vi "Waveform Shift 2 channels.vi"(8 "Trigger Info":cluster{"Trigger":bool, "Trig Offset":u8}, 9 "Input Valid":bool, 11 "Input Data":i16[](array[numeric])=[0, 0, 0, 0, 0, 0, 0, 0]) -> (0 "Trig Info":cluster{"Trigger":bool, "Trig Offset":u8}, 1 "Output Valid":bool, 3 "Shifted Output Data":i16[](array[numeric]), 4 "Trig Num":u8)   [LabVIEW 2012]
uses:
  <vilib>/rvi/FXPMathLib/basic elements/FxpDiscreteDelay/XNode/nifxpmath_DiscreteDelay.xnode
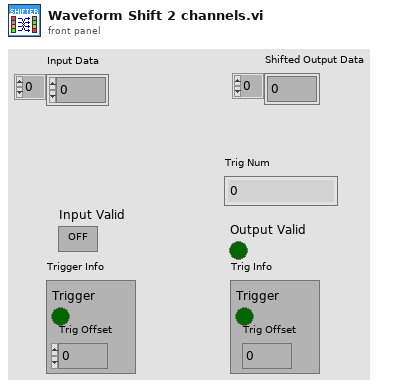
[diagram p1: front panel]
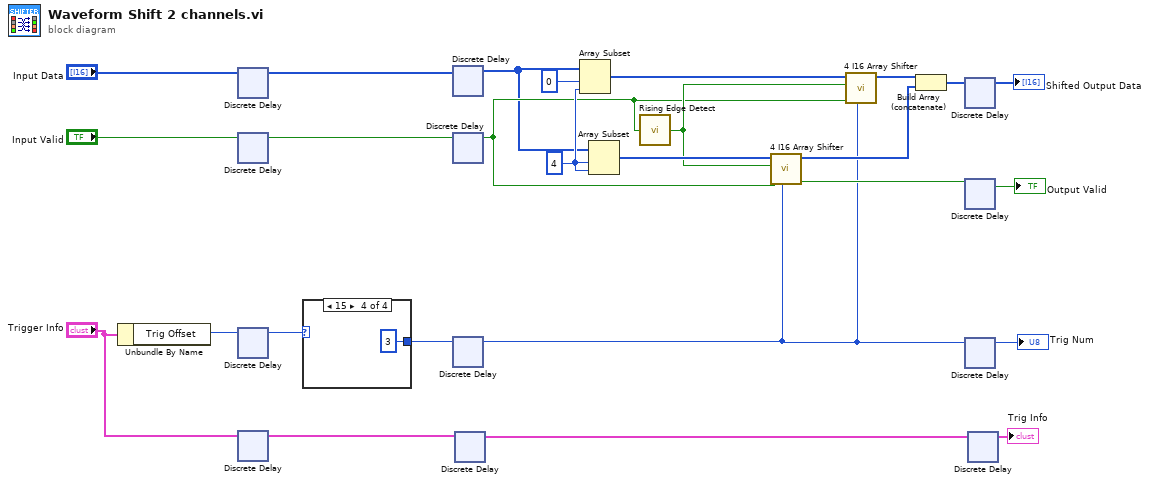
[diagram p0: block diagram]
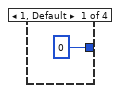
[diagram p2: hidden frame]
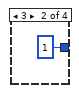
[diagram p3: hidden frame]
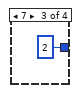
[diagram p4: hidden frame]
diagram:
  w26 = 4 ("index")
  n1 = Unbundle By Name("Trigger Info") -> ("Trig Offset"=w10:u8)
  n2 = xnode "Discrete Delay"("D"="Input Data") -> ("Q"=w6:i16[])
  n3 = xnode "Discrete Delay"("D"="Input Valid") -> ("Q"=w7:bool)
  n4 = xnode "Discrete Delay"("D"=w10) -> ("Q"=w3:u8)
  n5 = xnode "Discrete Delay"("D"="Trigger Info") -> ("Q"=w5:cluster{"Trigger":bool, "Trig Offset":u8})
  n6 = case shown="15" w3 {
    tunnel: [u8 0 u8 1 u8 2 u8 3] -> w2
    frame 1, Default {
    }
    frame 3 {
    }
    frame 7 {
    }
    frame 15 {
    }
  }
  n7 = xnode "Discrete Delay"("D"=w6) -> ("Q"=w17:i16[])
  n8 = xnode "Discrete Delay"("D"=w7) -> ("Q"=w18:bool)
  n9 = xnode "Discrete Delay"("D"=w2) -> ("Q"=w1:u8)
  n10 = xnode "Discrete Delay"("D"=w5) -> ("Q"=w9:cluster{"Trigger":bool, "Trig Offset":u8})
  n11 = Array Subset(array=w17, index=0, length=w26) -> (w16:i16[])
  n12 = Array Subset(array=w17, index=w26, length=w26) -> (w24:i16[])
  n13 = call <userlib>:"Rising Edge Detect.vi"("signal"=w18) -> ("edge detected"=w20:bool)  [unwired: 14 in]
  n14 = call <userlib>:"4 I16 Array Shifter.vi"("Trig Offset"=w1, "Input Valid"=w18, "Start of Read"=w20, "Input Data"=w24) -> ("Output Data Valid"=w19:bool, "Output Data"=w22:i16[])  [unwired: 6 in]
  n15 = call <userlib>:"4 I16 Array Shifter.vi"("Trig Offset"=w1, "Input Valid"=w18, "Start of Read"=w20, "Input Data"=w16) -> ("Output Data"=w23:i16[])  [unwired: 6 in, 1 out]
  n16 = Build Array (concatenate)(w23, w22) -> (w21:i16[])
  n17 = xnode "Discrete Delay"("D"=w21) -> ("Q"=→"Shifted Output Data":i16[])
  n18 = xnode "Discrete Delay"("D"=w19) -> ("Q"=→"Output Valid":bool)
  n19 = xnode "Discrete Delay"("D"=w1) -> ("Q"=→"Trig Num":u8)
  n20 = xnode "Discrete Delay"("D"=w9) -> ("Q"=→"Trig Info":cluster{"Trigger":bool, "Trig Offset":u8})
